vi "Read Message.vi"(6 "timeout ms (25000)":i32, 8 "error in (no error)":errorcluster, 11 "GenNet Protocol in":refnum<class "GenNet Protocol.lvclass">) -> (0 "error out":errorcluster, 2 "Message":variant, 3 "GenNet Protocol out":refnum<class "GenNet Protocol.lvclass">)   [LabVIEW 2020, in "hse-gennet.lvlib" / "GenNet Protocol.lvclass"]
doc: "____\nHAMPEL SOFTWARE ENGINEERING v3.8.0 (2023-12-18 14:41)"
uses:
  GenNet Protocol.lvclass
  GenNet Protocol.lvclass/GenNet Protocol.ctl
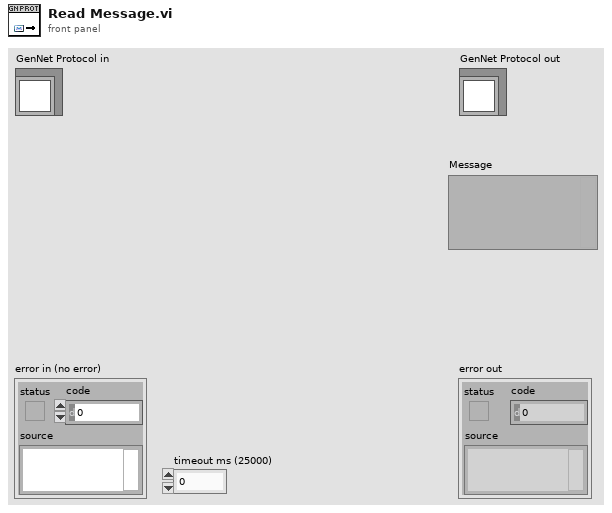
[diagram p1: front panel]
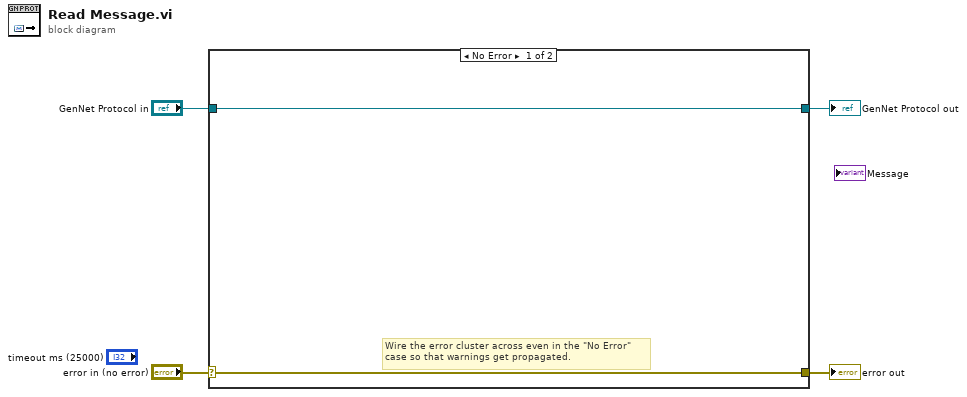
[diagram p0: block diagram]
diagram:
  n1 = case shown="No Error" "error in (no error)" {
    selector: "error in (no error)" -> [w5 w8]
    tunnel: [w5 w8] -> w3
    tunnel: [w6 w7] -> w1
    tunnel: "GenNet Protocol in" -> [w6 w7]
    frame No Error {
      # "Wire the error cluster across even in the \"No Error\"\ncase so that warnings get propagated."
    }
    frame Error {
    }
  }
  "error out" <- w3
  "GenNet Protocol out" <- w1
